vi "VI Tree.vi"   [LabVIEW 2020, in "IT-M3400.lvlib"]
doc: "This is the instrument driver for the <INSTRUMENT NAME>. The VI Tree displays all the user-callable VIs of the instrument driver in an organized table."
uses:
  IT-M3400.lvlib
panel:
  # "(c) 2014 <Enter Company Name Here>.  ALL RIGHTS RESERVED."
  # "SEE DIAGRAM\nFOR VI TREE."
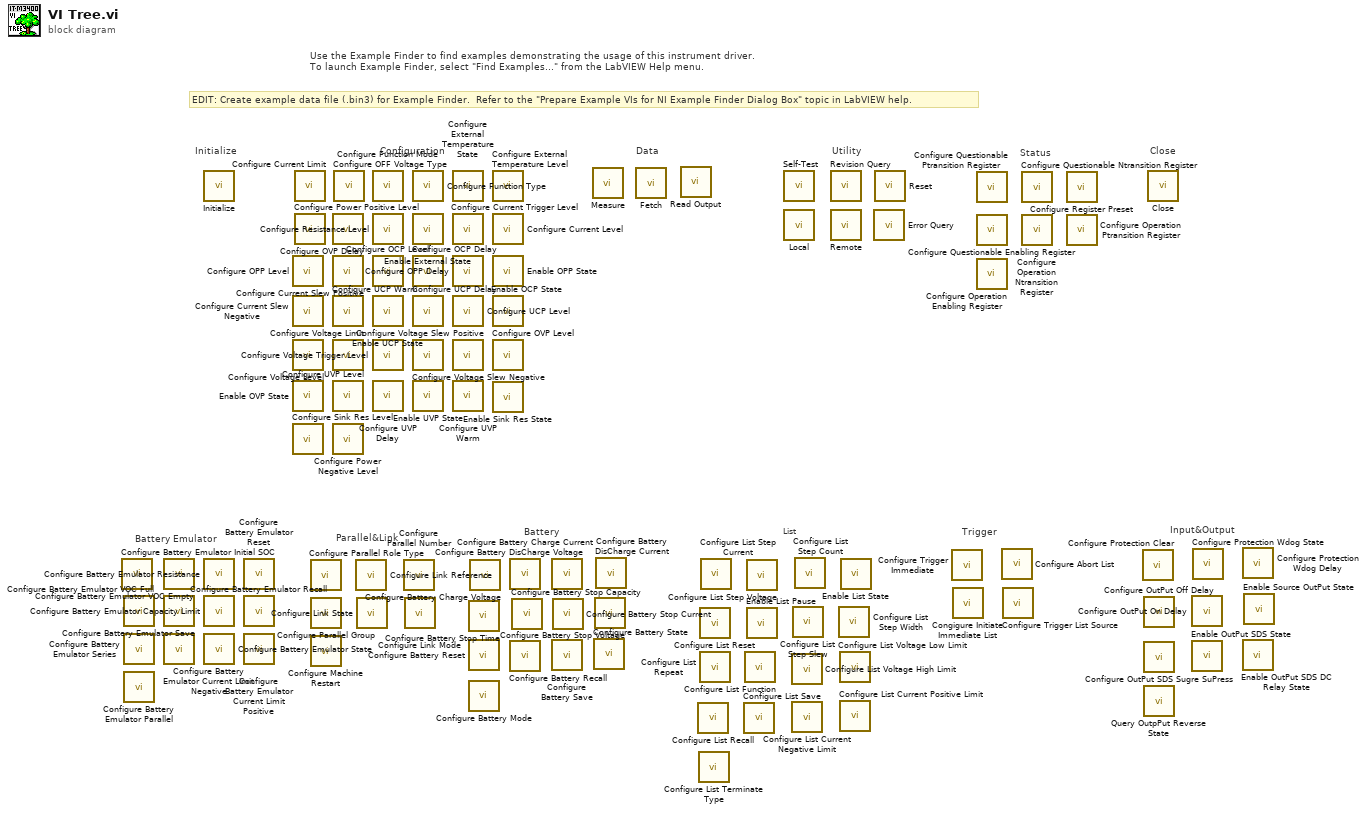
[diagram p0: block diagram]
diagram:
  # "Input&Output"
  # "Trigger"
  # "List"
  # "Battery"
  # "Parallel&Link"
  # "Battery Emulator"
  # "Status"
  # "EDIT: Create example data file (.bin3) for Example Finder.  Refer to the \"Prepare Example VIs for NI Example Finder Dialog Box\" topic in LabVIEW help."
  # "Use the Example Finder to find examples demonstrating the usage of this instrument driver.\nTo launch Example Finder, select \"Find Examples...\" from the LabVIEW Help menu."
  # "Configuration"
  # "Utility"
  # "Data"
  # "Close"
  # "Initialize"
  n1 = call "Configure Battery Emulator Initial SOC.vi"() -> ()  [unwired: 10 in, 2 out]
  n2 = call "Configure Battery Emulator VOC Full.vi"() -> ()  [unwired: 10 in, 2 out]
  n3 = call "Configure Battery Emulator Series.vi"() -> ()  [unwired: 10 in, 2 out]
  n4 = call "Configure Battery Emulator Parallel.vi"() -> ()  [unwired: 10 in, 2 out]
  n5 = call "Configure Battery Emulator VOC Empty.vi"() -> ()  [unwired: 10 in, 2 out]
  n6 = call "Configure Battery Emulator Save.vi"() -> ()  [unwired: 10 in, 2 out]
  n7 = call "Configure Battery Emulator Current Limit Negative.vi"() -> ()  [unwired: 10 in, 2 out]
  n8 = call <instrlib>:"Initialize.vi"() -> ()  [unwired: 10 in, 2 out]
  n9 = call "Configure Battery Emulator Resistance.vi"() -> ()  [unwired: 10 in, 2 out]
  n10 = call "Configure Battery Emulator Capacity Limit.vi"() -> ()  [unwired: 10 in, 2 out]
  n11 = call "Configure Battery Emulator State.vi"() -> ()  [unwired: 10 in, 2 out]
  n12 = call "Configure Battery Emulator Reset.vi"() -> ()  [unwired: 10 in, 2 out]
  n13 = call "Configure Battery Emulator Recall.vi"() -> ()  [unwired: 10 in, 2 out]
  n14 = call "Configure Battery Emulator Current Limit Positive.vi"() -> ()  [unwired: 10 in, 2 out]
  n15 = call "Configure OPP Level.vi"() -> ()  [unwired: 10 in, 2 out]
  n16 = call "Configure Current Slew Negative.vi"() -> ()  [unwired: 10 in, 2 out]
  n17 = call "Configure Voltage Level.vi"() -> ()  [unwired: 10 in, 2 out]
  n18 = call "Enable OVP State.vi"() -> ()  [unwired: 10 in, 2 out]
  n19 = call "Configure Sink Res Level.vi"() -> ()  [unwired: 10 in, 2 out]
  n20 = call "Configure Current Limit.vi"() -> ()  [unwired: 10 in, 2 out]
  n21 = call "Configure Power Positive Level.vi"() -> ()  [unwired: 10 in, 2 out]
  n22 = call "Configure Parallel Role Type.vi"() -> ()  [unwired: 10 in, 2 out]
  n23 = call "Configure Parallel Group.vi"() -> ()  [unwired: 10 in, 2 out]
  n24 = call "Configure Machine Restart.vi"() -> ()  [unwired: 10 in, 2 out]
  n25 = call "Configure OVP Delay.vi"() -> ()  [unwired: 10 in, 2 out]
  n26 = call "Configure Current Slew Positive.vi"() -> ()  [unwired: 10 in, 2 out]
  n27 = call "Configure UCP Warm.vi"() -> ()  [unwired: 10 in, 2 out]
  n28 = call "Configure Voltage Limit.vi"() -> ()  [unwired: 10 in, 2 out]
  n29 = call "Configure UVP Level.vi"() -> ()  [unwired: 10 in, 2 out]
  n30 = call "Configure Power Negative Level.vi"() -> ()  [unwired: 10 in, 2 out]
  n31 = call "Configure OFF Voltage Type.vi"() -> ()  [unwired: 10 in, 2 out]
  n32 = call "Configure Link Reference.vi"() -> ()  [unwired: 10 in, 2 out]
  n33 = call "Configure Link State.vi"() -> ()  [unwired: 10 in, 2 out]
  n34 = call "Configure Function Mode.vi"() -> ()  [unwired: 10 in, 2 out]
  n35 = call "Configure Resistance Level.vi"() -> ()  [unwired: 10 in, 2 out]
  n36 = call "Configure OCP Level.vi"() -> ()  [unwired: 10 in, 2 out]
  n37 = call "Enable UCP State.vi"() -> ()  [unwired: 10 in, 2 out]
  n38 = call "Configure Voltage Trigger Level.vi"() -> ()  [unwired: 10 in, 2 out]
  n39 = call "Configure UVP Delay.vi"() -> ()  [unwired: 10 in, 2 out]
  n40 = call "Configure Parallel Number.vi"() -> ()  [unwired: 10 in, 2 out]
  n41 = call "Configure Link Mode.vi"() -> ()  [unwired: 10 in, 2 out]
  n42 = call "Configure Function Type.vi"() -> ()  [unwired: 10 in, 2 out]
  n43 = call "Enable External State.vi"() -> ()  [unwired: 10 in, 2 out]
  n44 = call "Configure OCP Delay.vi"() -> ()  [unwired: 10 in, 2 out]
  n45 = call "Configure UCP Delay.vi"() -> ()  [unwired: 10 in, 2 out]
  n46 = call "Configure Voltage Slew Negative.vi"() -> ()  [unwired: 10 in, 2 out]
  n47 = call "Enable UVP State.vi"() -> ()  [unwired: 10 in, 2 out]
  n48 = call "Configure External Temperature State.vi"() -> ()  [unwired: 10 in, 2 out]
  n49 = call "Configure Current Trigger Level.vi"() -> ()  [unwired: 10 in, 2 out]
  n50 = call "Configure OPP Delay.vi"() -> ()  [unwired: 10 in, 2 out]
  n51 = call "Configure UCP Level.vi"() -> ()  [unwired: 10 in, 2 out]
  n52 = call "Configure Voltage Slew Positive.vi"() -> ()  [unwired: 10 in, 2 out]
  n53 = call "Configure UVP Warm.vi"() -> ()  [unwired: 10 in, 2 out]
  n54 = call "Configure Battery Stop Time.vi"() -> ()  [unwired: 10 in, 2 out]
  n55 = call "Configure Battery Reset.vi"() -> ()  [unwired: 10 in, 2 out]
  n56 = call "Configure Battery Mode.vi"() -> ()  [unwired: 10 in, 2 out]
  n57 = call "Configure Battery Charge Voltage.vi"() -> ()  [unwired: 9 in, 2 out]
  n58 = call "Configure External Temperature Level.vi"() -> ()  [unwired: 10 in, 2 out]
  n59 = call "Configure Current Level.vi"() -> ()  [unwired: 10 in, 2 out]
  n60 = call "Enable OPP State.vi"() -> ()  [unwired: 10 in, 2 out]
  n61 = call "Enable OCP State.vi"() -> ()  [unwired: 10 in, 2 out]
  n62 = call "Configure OVP Level.vi"() -> ()  [unwired: 10 in, 2 out]
  n63 = call "Enable Sink Res State.vi"() -> ()  [unwired: 10 in, 2 out]
  n64 = call "Configure Battery Charge Current.vi"() -> ()  [unwired: 10 in, 2 out]
  n65 = call "Configure Battery Recall.vi"() -> ()  [unwired: 10 in, 2 out]
  n66 = call "Configure Battery Stop Capacity.vi"() -> ()  [unwired: 10 in, 2 out]
  n67 = call "Configure Battery DisCharge Voltage.vi"() -> ()  [unwired: 10 in, 2 out]
  n68 = call "Configure Battery Save.vi"() -> ()  [unwired: 10 in, 2 out]
  n69 = call "Configure Battery Stop Current.vi"() -> ()  [unwired: 10 in, 2 out]
  n70 = call "Measure.vi"() -> ()  [unwired: 8 in, 3 out]
  n71 = call "Configure Battery State.vi"() -> ()  [unwired: 10 in, 2 out]
  n72 = call "Configure Battery Stop Voltage.vi"() -> ()  [unwired: 10 in, 2 out]
  n73 = call "Configure Battery DisCharge Current.vi"() -> ()  [unwired: 10 in, 2 out]
  n74 = call "Fetch.vi"() -> ()  [unwired: 9 in, 3 out]
  n75 = call <instrlib>:"Read Output.vi"() -> ()  [unwired: 8 in, 4 out]
  n76 = call "Configure List Recall.vi"() -> ()  [unwired: 10 in, 2 out]
  n77 = call "Configure List Terminate Type.vi"() -> ()  [unwired: 9 in, 2 out]
  n78 = call "Configure List Reset.vi"() -> ()  [unwired: 10 in, 2 out]
  n79 = call "Configure List Repeat.vi"() -> ()  [unwired: 10 in, 2 out]
  n80 = call "Configure List Step Current.vi"() -> ()  [unwired: 10 in, 2 out]
  n81 = call "Configure List Save.vi"() -> ()  [unwired: 10 in, 2 out]
  n82 = call "Configure List Function.vi"() -> ()  [unwired: 10 in, 2 out]
  n83 = call "Configure List Step Voltage.vi"() -> ()  [unwired: 10 in, 2 out]
  n84 = call "Enable List Pause.vi"() -> ()  [unwired: 10 in, 2 out]
  n85 = call "Self-Test.vi"() -> ()  [unwired: 8 in, 4 out]
  n86 = call "Local.vi"() -> ()  [unwired: 10 in, 2 out]
  n87 = call "Configure List Voltage High Limit.vi"() -> ()  [unwired: 10 in, 2 out]
  n88 = call "Configure List Current Negative Limit.vi"() -> ()  [unwired: 10 in, 2 out]
  n89 = call "Configure List Step Slew.vi"() -> ()  [unwired: 10 in, 2 out]
  n90 = call "Configure List Step Count.vi"() -> ()  [unwired: 10 in, 2 out]
  n91 = call "Revision Query.vi"() -> ()  [unwired: 8 in, 4 out]
  n92 = call "Remote.vi"() -> ()  [unwired: 10 in, 2 out]
  n93 = call "Configure List Step Width.vi"() -> ()  [unwired: 10 in, 2 out]
  n94 = call "Configure List Voltage Low Limit.vi"() -> ()  [unwired: 10 in, 2 out]
  n95 = call "Configure List Current Positive Limit.vi"() -> ()  [unwired: 10 in, 2 out]
  n96 = call "Enable List State.vi"() -> ()  [unwired: 10 in, 2 out]
  n97 = call <instrlib>:"Error Query.vi"() -> ()  [unwired: 8 in, 4 out]
  n98 = call "Reset.vi"() -> ()  [unwired: 10 in, 2 out]
  n99 = call "Configure Trigger Immediate.vi"() -> ()  [unwired: 10 in, 2 out]
  n100 = call "Congigure Initiate Immediate List.vi"() -> ()  [unwired: 10 in, 2 out]
  n101 = call "Configure Questionable Ptransition Register.vi"() -> ()  [unwired: 10 in, 2 out]
  n102 = call "Configure Questionable Enabling Register.vi"() -> ()  [unwired: 10 in, 2 out]
  n103 = call "Configure Operation Enabling Register.vi"() -> ()  [unwired: 10 in, 2 out]
  n104 = call "Configure Abort List.vi"() -> ()  [unwired: 10 in, 2 out]
  n105 = call "Configure Trigger List Source.vi"() -> ()  [unwired: 10 in, 2 out]
  n106 = call "Configure Questionable Ntransition Register.vi"() -> ()  [unwired: 10 in, 2 out]
  n107 = call "Configure Operation Ntransition Register.vi"() -> ()  [unwired: 10 in, 2 out]
  n108 = call "Configure Register Preset.vi"() -> ()  [unwired: 10 in, 2 out]
  n109 = call "Configure Operation Ptransition Register.vi"() -> ()  [unwired: 10 in, 2 out]
  n110 = call "Configure Protection Clear.vi"() -> ()  [unwired: 9 in, 2 out]
  n111 = call "Configure OutPut Off Delay.vi"() -> ()  [unwired: 10 in, 2 out]
  n112 = call "Configure OutPut SDS Sugre SuPress.vi"() -> ()  [unwired: 10 in, 2 out]
  n113 = call "Query OutpPut Reverse State.vi"() -> ()  [unwired: 9 in, 3 out]
  n114 = call <instrlib>:"Close.vi"() -> ()  [unwired: 11 in, 1 out]
  n115 = call "Configure OutPut On Delay.vi"() -> ()  [unwired: 10 in, 2 out]
  n116 = call "Enable OutPut SDS State.vi"() -> ()  [unwired: 10 in, 2 out]
  n117 = call "Configure Protection Wdog State.vi"() -> ()  [unwired: 10 in, 2 out]
  n118 = call "Configure Protection Wdog Delay.vi"() -> ()  [unwired: 10 in, 2 out]
  n119 = call "Enable OutPut SDS DC Relay State.vi"() -> ()  [unwired: 10 in, 2 out]
  n120 = call "Enable Source OutPut State.vi"() -> ()  [unwired: 10 in, 2 out]
